vi "main.vi"(10 "Output Path":path, 11 "Input Path":path) -> ()   [LabVIEW 2018]
uses:
  <vilib>/vision/NI_Vision_Development_Module.lvlib
panel:
  out "Converting File":dbl(slide) scale=0.0..100.0
  out "Image":T1(plugin-control)
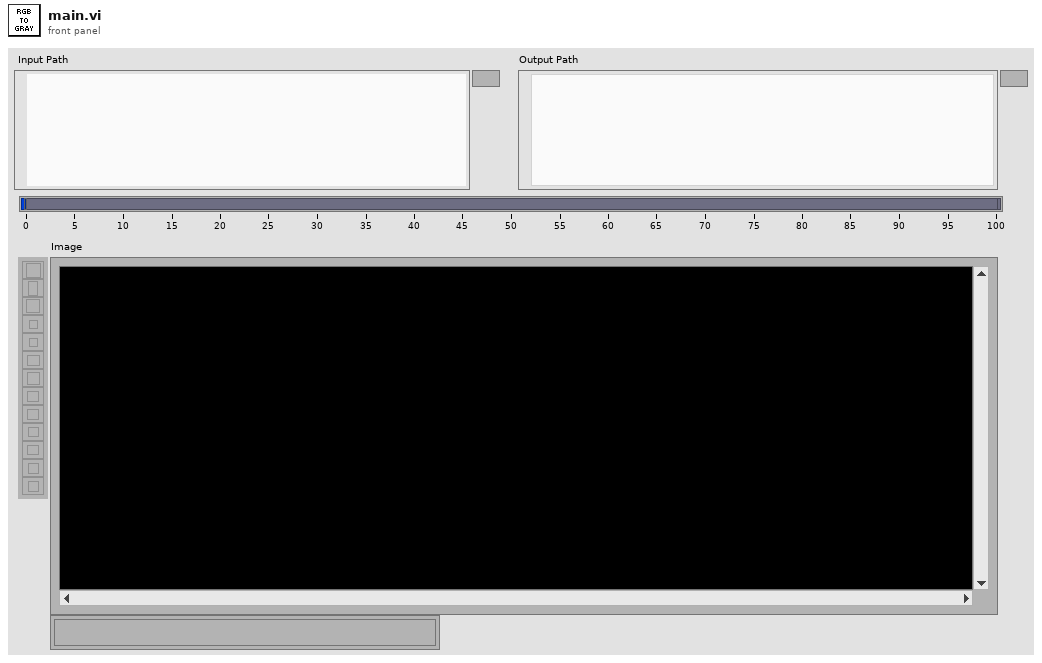
[diagram p1: front panel]
types:
  T1 = typedef "IMAQ Image.ctl" = refnum<image>
  T2 = typedef "Image Type" = u32
  T3 = typedef "IMAQ AVI2 Refnum.ctl" = refnum<k20>
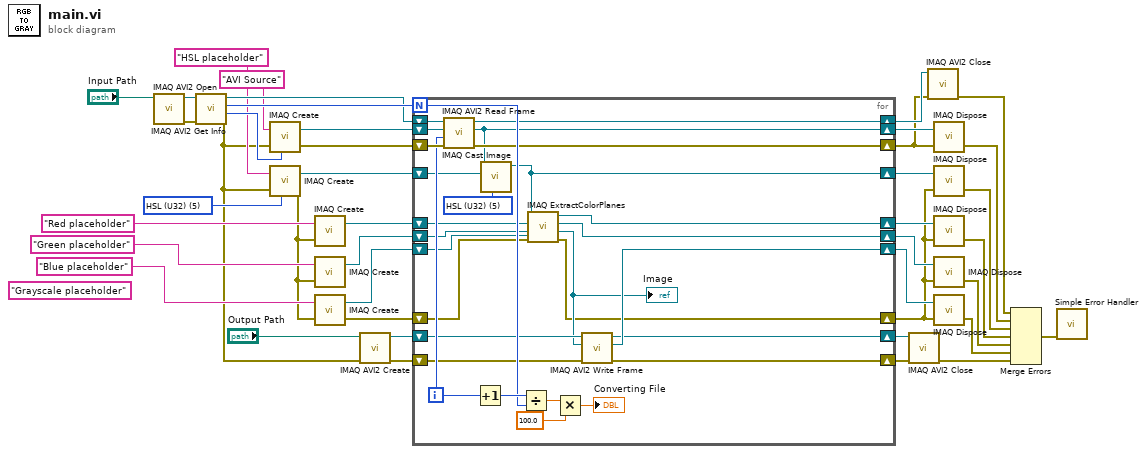
[diagram p0: block diagram]
diagram:
  (unwired) "Grayscale placeholder" ("Image Name")
  w28 = T2 5 items=["Grayscale (U8)", "Grayscale (I16)", "Grayscale (SGL)", "Complex (CSG)", "RGB (U32)", "HSL (U32)", "RGB (U64)", "Grayscale (U16)"] ("Image Type")
  n1 = call "IMAQ AVI2 Open"("AVI File Path"="Input Path") -> ("error out"=w40:errorcluster, "AVI Refnum"=w41:T3)  [unwired: 9 in]
  n2 = call "IMAQ AVI2 Get Info"("error in (no error)"=w40, "AVI Refnum"=w41) -> ("error out"=w12:errorcluster, "Image Type"=w36:T2, "Number of Frames"=w39:u32, "AVI Refnum (duplicate)"=w38:T3)  [unwired: 5 in, 1 out]
  n3 = call "IMAQ Create"("Image Name"="AVI Source", "Image Type"=w36, "error in (no error)"=w12) -> ("New Image"=w35:T1, "error out"=w34:errorcluster)  [unwired: 2 in]
  n4 = call "IMAQ Create"("Image Name"="HSL placeholder", "Image Type"=w28, "error in (no error)"=w12) -> ("New Image"=w29:T1, "error out"=w19:errorcluster)  [unwired: 2 in]
  n5 = call "IMAQ Create"("Image Name"="Red placeholder", "error in (no error)"=w19) -> ("New Image"=w27:T1)  [unwired: 3 in, 1 out]
  n6 = call "IMAQ Create"("Image Name"="Green placeholder", "error in (no error)"=w19) -> ("New Image"=w21:T1)  [unwired: 3 in, 1 out]
  n7 = call "IMAQ Create"("Image Name"="Blue placeholder", "error in (no error)"=w19) -> ("New Image"=w20:T1, "error out"=w16:errorcluster)  [unwired: 3 in]
  n8 = call "IMAQ AVI2 Create"("error in (no error)"=w12, "AVI Path"="Output Path") -> ("error out"=w11:errorcluster, "AVI Refnum"=w14:T3)  [unwired: 8 in]
  n9 = for {
    N: w39 -> [w69]
    shift-right: [w61] -> w33
    shift-left: w38 -> [w65]
    shift-right: [w59] -> w32
    shift-left: w35 -> [w64]
    shift-right: [w60] -> w31
    shift-left: w34 -> [w63]
    shift-right: [w56] -> w26
    shift-left: w29 -> [w58]
    shift-right: [w52] -> w25
    shift-left: w27 -> [w55]
    shift-right: [w51] -> w18
    shift-left: w21 -> [w54]
    shift-right: [w47] -> w17
    shift-left: w20 -> [w53]
    shift-right: [w43] -> w15
    shift-left: w16 -> [w50]
    shift-right: [w45] -> w9
    shift-left: w11 -> [w48]
    shift-right: [w46] -> w10
    shift-left: w14 -> [w49]
    i -> [w62]
    w57 = T2 5 items=["Grayscale (U8)", "Grayscale (I16)", "Grayscale (SGL)", "Complex (CSG)", "RGB (U32)", "HSL (U32)", "RGB (U64)", "Grayscale (U16)"] ("Image Type")
    n10 = call "IMAQ AVI2 Read Frame"("error in (no error)"=w63, "Frame Number"=w62, "Image"=w64, "AVI Refnum"=w65) -> ("error out"=w60:errorcluster, "Image Out"=w59:T1, "AVI Refnum (duplicate)"=w61:T3)  [unwired: 5 in]
    n11 = Increment(x=w62) -> (x+1=w70:i32)
    n12 = call "IMAQ Cast Image"("Image Type"=w57, "Image Dst"=w58, "Image Src"=w59) -> ("Image Dst Out"=w56:T1)  [unwired: 7 in, 1 out]
    n13 = Divide(x=w70, y=w69) -> (x/y=w68:dbl)
    n14 = call "IMAQ ExtractColorPlanes"("Blue or Luma or Val or Inten Plane"=w53, "error in (no error)"=w50, "Green or Sat Plane"=w54, "Red or Hue Plane"=w55, "Image Src"=w56) -> ("error out"=w43:errorcluster, "Blue or Luma or Val or Inten Plane out"=w44:T1, "Green or Sat Plane out"=w51:T1, "Red or Hue Plane out"=w52:T1)  [unwired: 3 in]
    "Image" <- w44
    n15 = Multiply(x=w68, y=100.0) -> (x*y=→"Converting File":dbl)
    n16 = call "IMAQ AVI2 Write Frame"("error in (no error)"=w48, "Image"=w44, "AVI Refnum"=w49) -> ("error out"=w45:errorcluster, "Image Out (duplicate)"=w47:T1, "AVI Refnum (duplicate)"=w46:T3)  [unwired: 6 in]
  }
  n17 = call "IMAQ AVI2 Close"("error in (no error)"=w9, "AVI Refnum"=w10) -> ("error out"=w8:errorcluster)  [unwired: 9 in]
  n18 = call "IMAQ AVI2 Close"("error in (no error)"=w31, "AVI Refnum"=w33) -> ("error out"=w2:errorcluster)  [unwired: 9 in]
  n19 = call "IMAQ Dispose"("Image"=w32, "error in (no error)"=w31) -> ("error out"=w3:errorcluster)  [unwired: 4 in]
  n20 = call "IMAQ Dispose"("Image"=w26, "error in (no error)"=w15) -> ("error out"=w4:errorcluster)  [unwired: 4 in]
  n21 = call "IMAQ Dispose"("Image"=w25, "error in (no error)"=w15) -> ("error out"=w5:errorcluster)  [unwired: 4 in]
  n22 = call "IMAQ Dispose"("Image"=w18, "error in (no error)"=w15) -> ("error out"=w6:errorcluster)  [unwired: 4 in]
  n23 = call "IMAQ Dispose"("Image"=w17, "error in (no error)"=w15) -> ("error out"=w7:errorcluster)  [unwired: 4 in]
  n24 = Merge Errors(w2, w3, w4, w5, w6, w7, w8) -> (w1:errorcluster)
  n25 = call <vilib>:"Simple Error Handler.vi"("error in (no error)"=w1) -> ()  [unwired: 4 in, 5 out]
